vi "processControls.vi"(8 "error in (no error)":errorcluster, 9 "Controls[]":refnum<vi>[](array[refnum]), 10 "Calling VI Reference i":refnum<vi>, 11 "Dependency in":refnum<class "Dependency.lvclass">) -> (0 "error out":errorcluster, 2 "Calling VI Reference o":refnum<vi>, 3 "Dependency out":refnum<class "Dependency.lvclass">)   [LabVIEW 2016, in "Dependency.lvclass"]
uses:
  Dependency.lvclass
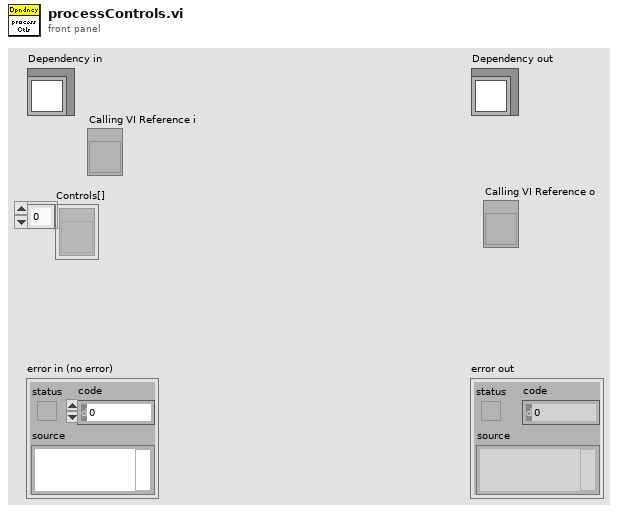
[diagram p1: front panel]
types:
  T1 = enum32{"not a typedef", "typedef", "strict typedef", "class private data"}
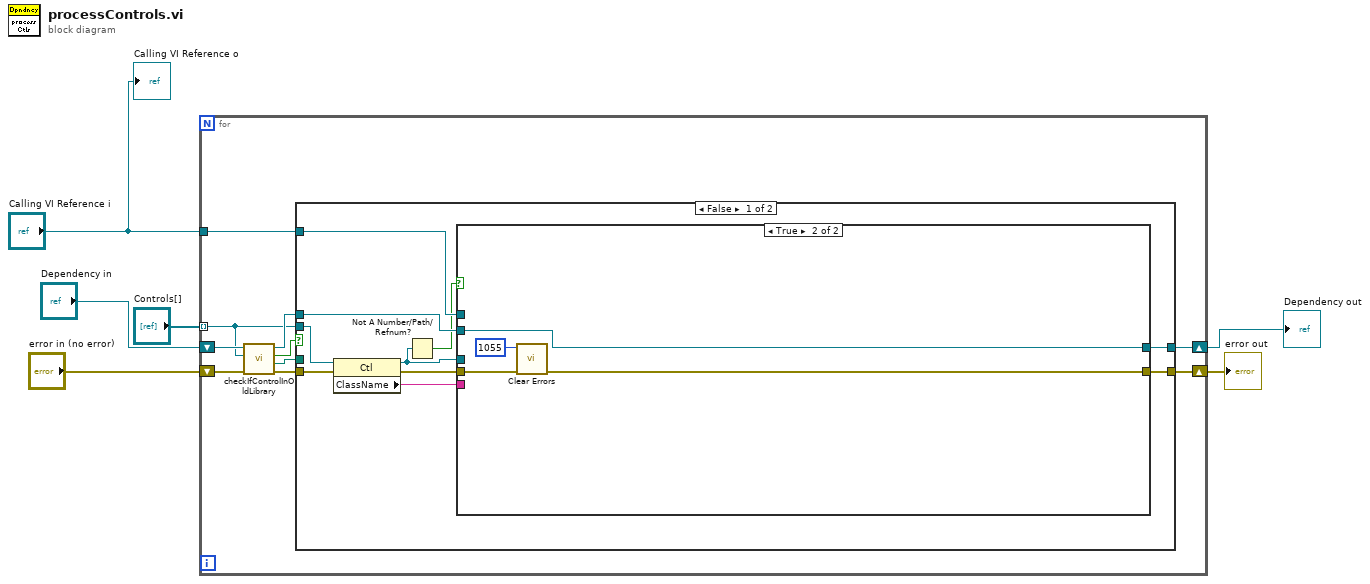
[diagram p0: block diagram]
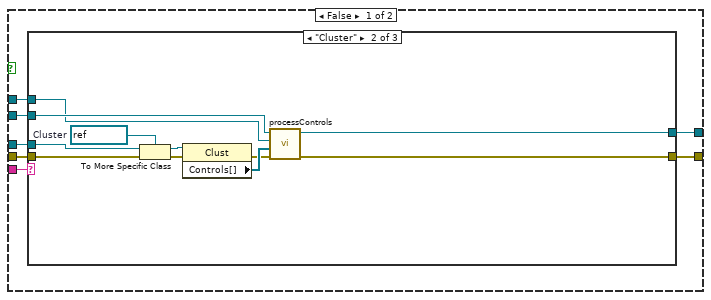
[diagram p2: hidden frame]
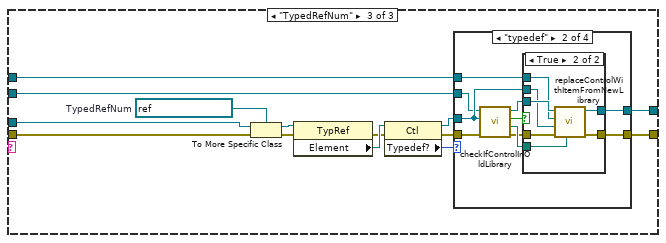
[diagram p4: hidden frame]
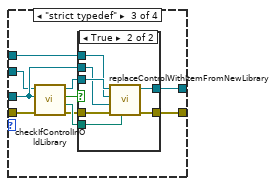
[diagram p7: hidden frame]
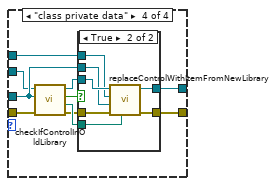
[diagram p9: hidden frame]
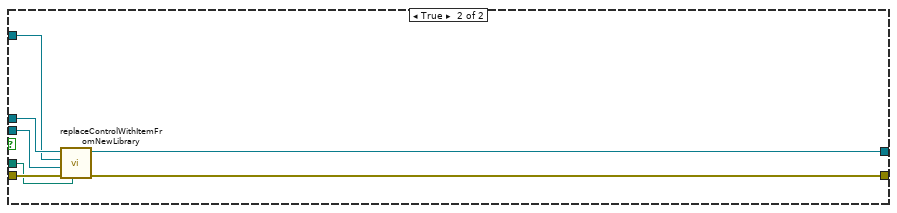
[diagram p11: hidden frame]
diagram:
  n1 = for {
    shift-right: [w10] -> w4
    shift-left: "Dependency in" -> [w16]
    tunnel: "Calling VI Reference i" -> [w9]
    tunnel: "Controls[]" -> [w11] mode=indexing
    shift-right: [w7] -> w2
    shift-left: "error in (no error)" -> [w13]
    n2 = call "checkIfControlInOldLibrary.vi"("error in (no error)"=w13, "Ctl Refnum"=w11, "Dependency in"=w16) -> ("error out"=w12:errorcluster, "CtrlPath"=w8:path, "isMemberOfOldLibrary"=w14:bool, "Dependency out"=w15:refnum<class "Dependency.lvclass">)  [unwired: 5 in]
    n3 = case shown="False" w14 {
      tunnel: w15 -> [w22 w130]
      tunnel: [w21 w129] -> w10
      tunnel: w9 -> [w23 w126]
      tunnel: w11 -> [w24 w128]
      tunnel: w12 -> [w20 w127]
      tunnel: [w19 w125] -> w7
      tunnel: w8 -> [_ w124]
      frame False {
        n4 = property class="Ctl"(reference=w24, error in=w20) -> (reference out=w18:refnum<vi>, error out=w25:errorcluster, "ClassName"=w26:string)
        n5 = Not A Number/Path/Refnum?(number/path/refnum=w18) -> (NaN/Path/Refnum?=w17:bool)
        n6 = case shown="True" w17 {
          tunnel: w26 -> [w33 _]
          tunnel: w25 -> [w32 w122]
          tunnel: w23 -> [w31 _]
          tunnel: w22 -> [w30 w120]
          tunnel: [w29 w120] -> w21
          tunnel: [w28 w121] -> w19
          tunnel: w18 -> [w27 _]
          frame False {
            n7 = case shown="\"Cluster\"" w33 {
              tunnel: w27 -> [_ w46 w59]
              tunnel: w30 -> [w35 w43 w55]
              tunnel: [w35 w42 w52] -> w29
              tunnel: w31 -> [_ w40 w54]
              tunnel: w32 -> [w34 w39 w51]
              tunnel: [w34 w36 w47] -> w28
              frame Default {
              }
              frame "Cluster" {
                w45 = refnum<vi> refnum  # Cluster
                n8 = To More Specific Class(target class=w45, reference=w46, error in=w39) -> (specific class reference=w44:refnum<vi>, error out=w38:errorcluster)
                n9 = property class="Clust"(reference=w44, error in=w38) -> (error out=w37:errorcluster, "Controls[]"=w41:refnum<vi>[])  [unwired: 1 out]
                n10 = call "processControls.vi"("error in (no error)"=w37, "Controls[]"=w41, "Calling VI Reference i"=w40, "Dependency in"=w43) -> ("error out"=w36:errorcluster, "Dependency out"=w42:refnum<class "Dependency.lvclass">)  [unwired: 5 in, 1 out]
              }
              frame "TypedRefNum" {
                w60 = refnum<vi> refnum  # TypedRefNum
                n11 = To More Specific Class(target class=w60, reference=w59, error in=w51) -> (specific class reference=w58:refnum<vi>, error out=w50:errorcluster)
                n12 = property class="TypRef"(reference=w58, error in=w50) -> (error out=w49:errorcluster, "Element"=w57:refnum<vi>)  [unwired: 1 out]
                n13 = property class="Ctl"(reference=w57, error in=w49) -> (reference out=w53:refnum<vi>, error out=w48:errorcluster, "Typedef?"=w56:T1)
                n14 = case shown="\"typedef\"" w56 {
                  tunnel: w55 -> [w62 w68 w87 w106]
                  tunnel: w54 -> [_ w72 w91 w110]
                  tunnel: w53 -> [_ w70 w89 w108]
                  tunnel: [w62 w69 w88 w107] -> w52
                  tunnel: w48 -> [w61 w65 w84 w103]
                  tunnel: [w61 w63 w82 w101] -> w47
                  frame "not a typedef", Default {
                  }
                  frame "typedef" {
                    n15 = call "checkIfControlInOldLibrary.vi"("error in (no error)"=w65, "Ctl Refnum"=w70, "Dependency in"=w68) -> ("error out"=w64:errorcluster, "CtrlPath"=w66:path, "isMemberOfOldLibrary"=w71:bool, "Dependency out"=w67:refnum<class "Dependency.lvclass">)  [unwired: 5 in]
                    n16 = case shown="True" w71 {
                      tunnel: w67 -> [w74 w81]
                      tunnel: w72 -> [_ w80]
                      tunnel: w70 -> [_ w79]
                      tunnel: w66 -> [_ w78]
                      tunnel: [w74 w77] -> w69
                      tunnel: w64 -> [w73 w76]
                      tunnel: [w73 w75] -> w63
                      frame False {
                      }
                      frame True {
                        n17 = call "replaceControlWithItemFromNewLibrary.vi"("SubVI Path"=w78, "error in (no error)"=w76, "Ctl Refnum"=w79, "Calling VI Reference"=w80, "Dependency in"=w81) -> ("error out"=w75:errorcluster, "Dependency out"=w77:refnum<class "Dependency.lvclass">)  [unwired: 5 in]
                      }
                    }
                  }
                  frame "strict typedef" {
                    n18 = call "checkIfControlInOldLibrary.vi"("error in (no error)"=w84, "Ctl Refnum"=w89, "Dependency in"=w87) -> ("error out"=w83:errorcluster, "CtrlPath"=w85:path, "isMemberOfOldLibrary"=w90:bool, "Dependency out"=w86:refnum<class "Dependency.lvclass">)  [unwired: 5 in]
                    n19 = case shown="True" w90 {
                      tunnel: w86 -> [w93 w100]
                      tunnel: w91 -> [_ w99]
                      tunnel: w89 -> [_ w98]
                      tunnel: w85 -> [_ w97]
                      tunnel: [w93 w96] -> w88
                      tunnel: w83 -> [w92 w95]
                      tunnel: [w92 w94] -> w82
                      frame False {
                      }
                      frame True {
                        n20 = call "replaceControlWithItemFromNewLibrary.vi"("SubVI Path"=w97, "error in (no error)"=w95, "Ctl Refnum"=w98, "Calling VI Reference"=w99, "Dependency in"=w100) -> ("error out"=w94:errorcluster, "Dependency out"=w96:refnum<class "Dependency.lvclass">)  [unwired: 5 in]
                      }
                    }
                  }
                  frame "class private data" {
                    n21 = call "checkIfControlInOldLibrary.vi"("error in (no error)"=w103, "Ctl Refnum"=w108, "Dependency in"=w106) -> ("error out"=w102:errorcluster, "CtrlPath"=w104:path, "isMemberOfOldLibrary"=w109:bool, "Dependency out"=w105:refnum<class "Dependency.lvclass">)  [unwired: 5 in]
                    n22 = case shown="True" w109 {
                      tunnel: w105 -> [w112 w119]
                      tunnel: w110 -> [_ w118]
                      tunnel: w108 -> [_ w117]
                      tunnel: w104 -> [_ w116]
                      tunnel: [w112 w115] -> w107
                      tunnel: w102 -> [w111 w114]
                      tunnel: [w111 w113] -> w101
                      frame False {
                      }
                      frame True {
                        n23 = call "replaceControlWithItemFromNewLibrary.vi"("SubVI Path"=w116, "error in (no error)"=w114, "Ctl Refnum"=w117, "Calling VI Reference"=w118, "Dependency in"=w119) -> ("error out"=w113:errorcluster, "Dependency out"=w115:refnum<class "Dependency.lvclass">)  [unwired: 5 in]
                      }
                    }
                  }
                }
              }
            }
          }
          frame True {
            n24 = call <vilib>:"Clear Errors.vi"("error in (no error)"=w122, "specific error code to clear (0: all)"=1055) -> ("error out"=w121:errorcluster)  [unwired: 4 in, 1 out]
          }
        }
      }
      frame True {
        n25 = call "replaceControlWithItemFromNewLibrary.vi"("SubVI Path"=w124, "error in (no error)"=w127, "Ctl Refnum"=w128, "Calling VI Reference"=w126, "Dependency in"=w130) -> ("error out"=w125:errorcluster, "Dependency out"=w129:refnum<class "Dependency.lvclass">)  [unwired: 5 in]
      }
    }
  }
  "error out" <- w2
  "Dependency out" <- w4
  "Calling VI Reference o" <- "Calling VI Reference i"
